vi "checkQR (SubVI).vi"(10 "Image Type":T1 items=["Grayscale (U8)", "Grayscale (I16)", "Grayscale (SGL)", "Complex (CSG)", "RGB (U32)", "HSL (U32)", "RGB (U64)", "Grayscale (U16)"], 11 "Refnum in":T2) -> (0 "error out":errorcluster, 1 "error out":errorcluster, 2 "Quantity:":i32, 3 "Refnum out":T3(plugin-control), 4 "Data":string, 5 "Mass (kg):":dbl, 6 "Tong K/lg (kg)":dbl, 7 "Found?":bool)   [LabVIEW 2015]
uses:
  <vilib>/userdefined/High Color/IMAQdx.ctl
  <vilib>/regexp/Match Regular Expression.xnode
  <vilib>/vision/driver/NI_Vision_Acquisition_Software.lvlib
  <vilib>/vision/NI_Vision_Development_Module.lvlib
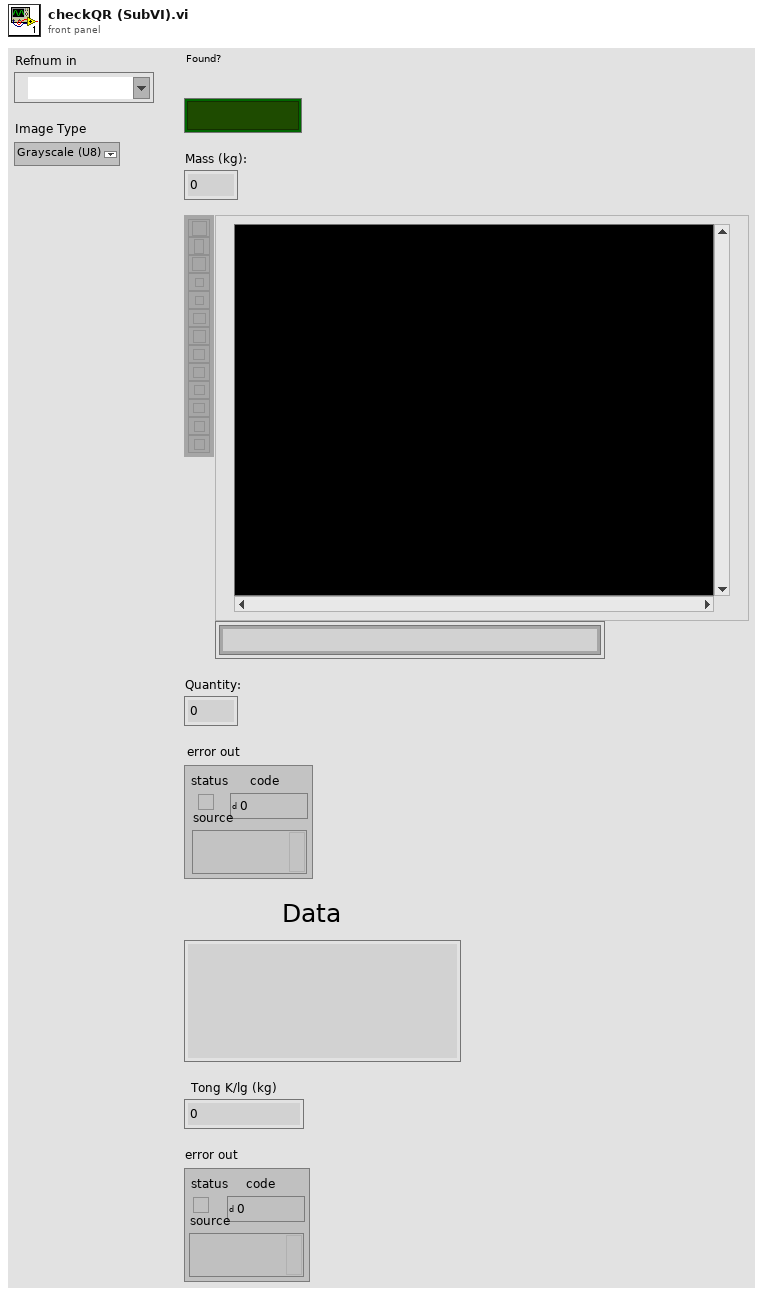
[diagram p1: front panel]
types:
  T1 = typedef "Image Type" = u32
  T2 = typedef "IMAQdx.ctl" = refnum<k21>
  T3 = typedef "IMAQ Image.ctl" = refnum<image>
  T4 = typedef "QR Code Report.ctl" = cluster{"Found?":bool, "Data":string, "Bounding Box":cluster{"x":sgl, "y":sgl}[], "Errors Corrected":u32, "Dimensions (Rows/Cols)":u32, "Version":u32, "QR Model":T5, "Stream Mode":T6, "Barcode Polarity":T7, "Mirrored?":bool, "Append Stream Position":u32, "Size of Append Stream":u32, "First EAN-128 ID":i32, "First Alternate Language ID":i32, "Append Stream ID":u32, "Minimum Edge Strength":u32, "Demodulation Mode":T8, "Cell Sample Size":T9, "Cell Filter Mode":T10}
  T5 = typedef "QR Code Model Type.ctl" = i32
  T6 = typedef "QR Code Stream Mode Type.ctl" = i32
  T7 = typedef "Data Matrix Polarity.ctl" = i32
  T8 = typedef "Demodulation Mode.ctl" = i32
  T9 = typedef "Cell Sample Size.ctl" = i32
  T10 = typedef "Cell Filter Mode.ctl" = i32
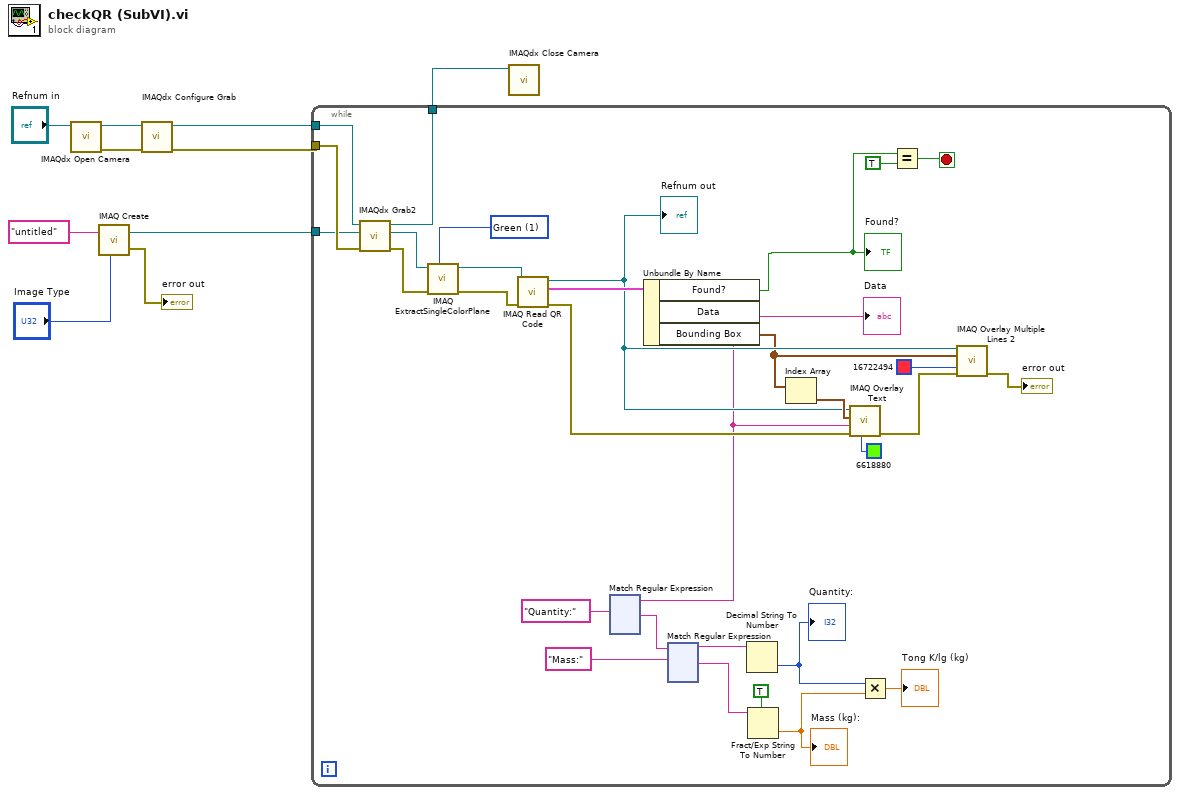
[diagram p0: block diagram]
diagram:
  n1 = call <vilib>:"IMAQdx Open Camera.vi"("Session In"="Refnum in") -> ("error out"=w6:errorcluster, "Session Out"=w5:T2)  [unwired: 9 in]
  n2 = call "IMAQ Create"("Image Name"="untitled", "Image Type"="Image Type") -> ("New Image"=w9:T3, "error out"=→"error out":errorcluster)  [unwired: 3 in]
  n3 = call <vilib>:"IMAQdx Configure Grab.vi"("error in"=w6, "Session In"=w5) -> ("error out"=w4:errorcluster, "Session Out"=w3:T2)  [unwired: 8 in]
  n4 = while {
    tunnel: [w41] -> w2
    tunnel: w3 -> [w40]
    tunnel: w4 -> [w39]
    tunnel: w9 -> [w38]
    stop <- w12 stop-if-true
    w34 = 1 items=["Red", "Green", "Blue", "Hue", "Saturation", "Luminance", "Value", "Intensity"] ("Color Plane")
    n5 = call <vilib>:"IMAQdx Grab2.vi"("error in"=w39, "Image In"=w38, "Session In"=w40) -> ("error out"=w35:errorcluster, "Image Out"=w36:T3, "Session Out"=w41:T2)  [unwired: 5 in, 1 out]
    n6 = call "IMAQ ExtractSingleColorPlane"("Color Plane"=w34, "error in (no error)"=w35, "Image Src"=w36) -> ("error out"=w37:errorcluster, "Image Dst Out"=w23:T3)  [unwired: 7 in]
    n7 = call "IMAQ Read QR Code"("error in (no error)"=w37, "Image"=w23) -> ("error out"=w25:errorcluster, "QR Code Report"=w33:T4, "Image (duplicate)"=w30:T3)  [unwired: 6 in, 1 out]
    "Refnum out" <- w30
    n8 = Unbundle By Name(w33) -> ("Found?"=w11:bool, "Data"=w21:string, "Bounding Box"=w29:cluster{"x":sgl, "y":sgl}[])
    "Found?" <- w11
    "Data" <- w21
    n9 = xnode "Match Regular Expression"("input string"=w21, "regular expression"="Quantity:") -> ("after match"=w19:string)  [unwired: 4 in, 4 out]
    n10 = xnode ("Match Regular Expression")("input string"=w19, "regular expression"="Mass:" ("regular expression 2")) -> ("before match"=w18:string, "after match"=w15:string)  [unwired: 4 in, 3 out]
    n11 = Decimal String To Number(string=w18) -> (number=w16:i32)  [unwired: 2 in, 1 out]
    "Quantity:" <- w16
    n12 = Fract/Exp String To Number(use system decimal point (T)=TRUE, string=w15) -> (number=w13:dbl)  [unwired: 2 in, 1 out]
    "Mass (kg):" <- w13
    n13 = Index Array(array=w29) -> (element=w32:cluster{"x":sgl, "y":sgl})  [unwired: 1 in]
    n14 = call "IMAQ Overlay Text"("Text Color (black)"=u32 6618880, "error in (no error)"=w25, "String"=w21, "Origin"=w32, "Image"=w30) -> ("error out"=w27:errorcluster)  [unwired: 5 in, 1 out]
    n15 = Multiply(x=w16, y=w13) -> (x*y=→"Tong K/lg (kg)":dbl)
    n16 = Equal?(x=w11, y=TRUE) -> (x = y?=w12:bool)
    n17 = call "IMAQ Overlay Multiple Lines 2"("Image"=w30, "Line End Points"=w29, "Color"=u32 16722494, "error in (no error)"=w27) -> ("error out"=→"error out":errorcluster)  [unwired: 10 in, 1 out]
  }
  n18 = call <vilib>:"IMAQdx Close Camera.vi"("Session In"=w2) -> ()  [unwired: 10 in, 1 out]
